vi "SOC_FM DotNet_MessageDialog.vi"(11 "info":string[](array[string])=["Signal Mean", "12.00", "Signal RMS", "10.1"]) -> ()   [LabVIEW 2014]
uses:
  E:/Files/subversion/C3/NIWeek/SepOfConcerns/Source/SOC_FM/subVIs/ClientDialogs.dll
  ClientDialogs.dll
panel:
  out "error out":errorcluster
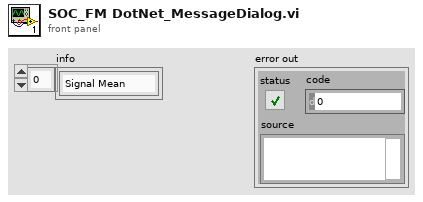
[diagram p1: front panel]
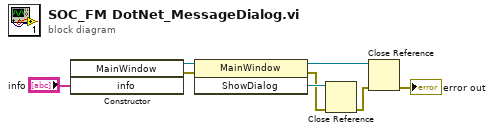
[diagram p0: block diagram]
diagram:
  n1 = constructor class="MainWindow"("info"="info") -> (reference out=w8:refnum<k24>, error out=w6:errorcluster)  [unwired: 3 in, 2 out]
  n2 = invoke class="MainWindow" method="ShowDialog"(reference=w8, error in=w6) -> (reference out=w7:refnum<k24>, error out=w3:errorcluster, "ShowDialog"=w4:refnum<k24>)  [unwired: 1 in]
  n3 = Close Reference(reference=w4, error in (no error)=w3) -> (error out=w2:errorcluster)
  n4 = Close Reference(reference=w7, error in (no error)=w2) -> (error out=→"error out":errorcluster)
